vi "Check_with_Jump.vi"(0 "Current position":dbl[](array[numeric])=[0.0, 200.0, 40.0] format="%.2f", 1 "Traverse Name":string, 3 "Simulate/Run":T2=enum."Run VI", 5 "New Position":dbl[](array[numeric])=[0.0, 100.0, 40.0] format="%.2f", 7 "Probe Support":T1=[{"Max"=10.0, "Min"=-10.0}, {"Max"=10.0, "Min"=-10.0}, {"Max"=200.0, "Min"=0.0}] {"Min" format="%#.1f"; "Max" format="%#.1f"}, 9 "Entire Space":T1=[{"Max"=500.0, "Min"=-500.0}, {"Max"=1000.0, "Min"=-1000.0}, {"Max"=700.0, "Min"=0.0}] {"Min" format="%#.1f"; "Max" format="%#.1f"}, 11 "Probe Volume":T1=[{"Max"=10.0, "Min"=-10.0}, {"Max"=10.0, "Min"=-10.0}, {"Max"=200.0, "Min"=0.0}] {"Min" format="%#.1f"; "Max" format="%#.1f"}, 13 "Exclude Array":T3[](array[typedef])=[{"Sizes"=[{"Max"=1000.0, "Min"=-1000.0}, {"Max"=1000.0, "Min"=-1000.0}, {"Max"=20.0, "Min"=0.0}], "Name"="Roughness Elements", "Exclude Type"=enum."Allow only vertical moves"}, {"Sizes"=[{"Max"=50.0, "Min"=-50.0}, {"Max"=50.0, "Min"=-50.0}, {"Max"=220.0, "Min"=-0.0}], "Name"="B204", "Exclude Type"=enum."Exclude completely"}] {"Sizes"."Min" format="%#.1f"; "Sizes"."Max" format="%#.1f"}, 14 "Model       Roll      Pitch       Yaw (deg)":dbl[](array[numeric]) format="%#.2f") -> (4 "Error Comments":string, 10 "Steps":dbl[][](array[numeric])=[[0.0, 200.0, 40.0]] format="%.2f")   [LabVIEW 2013]
uses:
  Box_size.ctl
  Exclude_cluster.ctl
  Exclusion_type.ctl
  Controls/User_Specific_mode.ctl
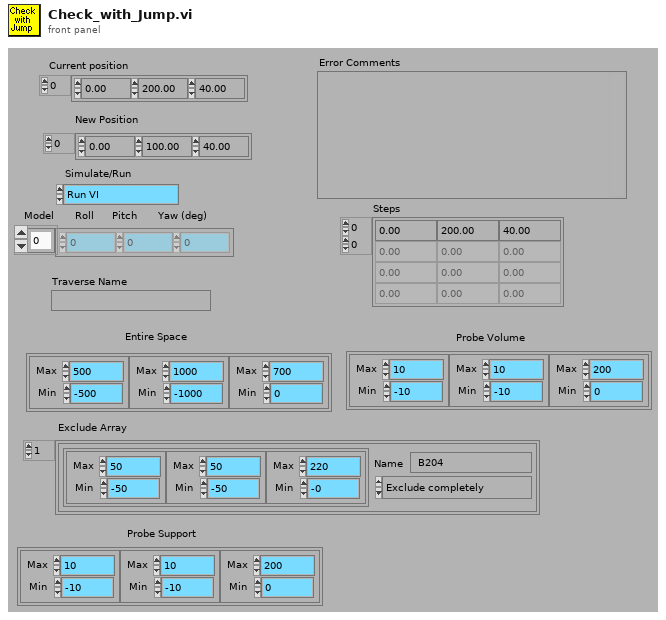
[diagram p1: front panel]
types:
  T1 = typedef "Box_size.ctl" = cluster{"Max":dbl, "Min":dbl}[]
  T2 = typedef "User_Specific_mode.ctl" = enum16{"Check VI only", "Run VI"}
  T3 = typedef "Exclude_cluster.ctl" = cluster{"Sizes":T1, "Name":string, "Exclude Type":T4}
  T4 = typedef "Exclusion_type.ctl" = enum16{"Exclude completely", "Allow only vertical moves"}
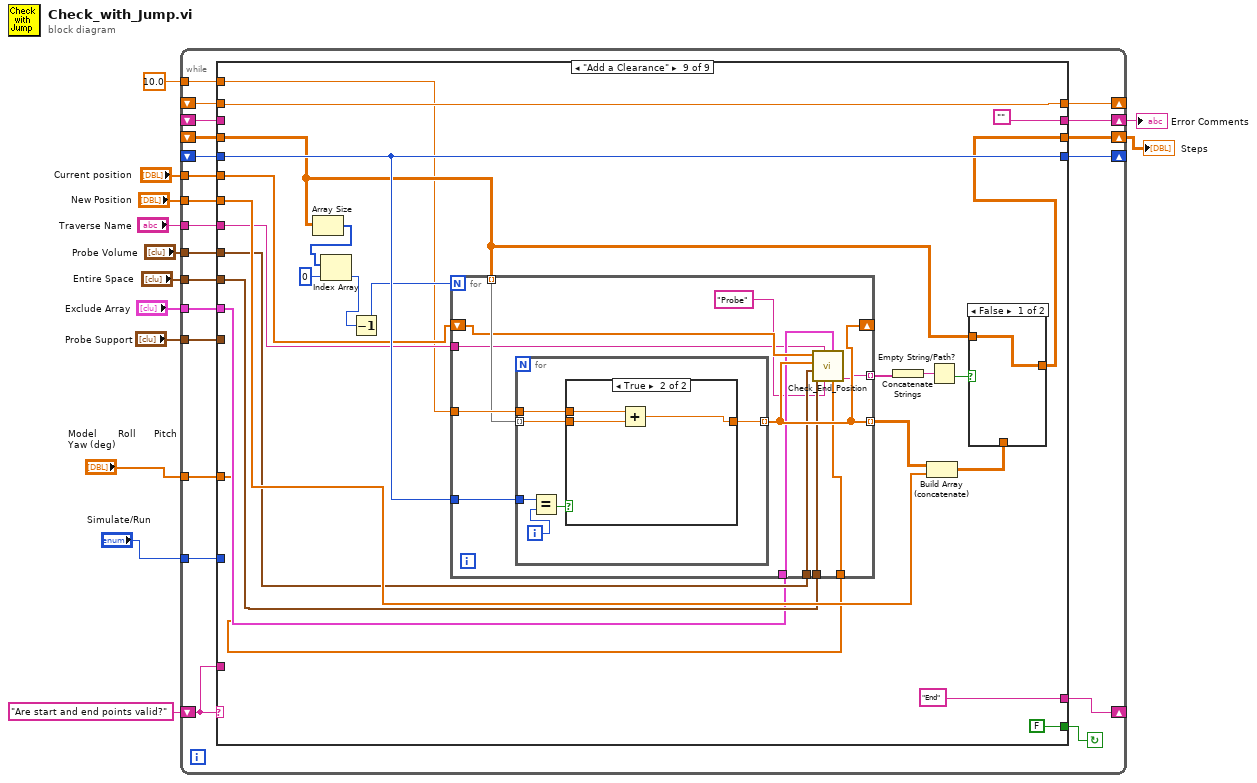
[diagram p0: block diagram]
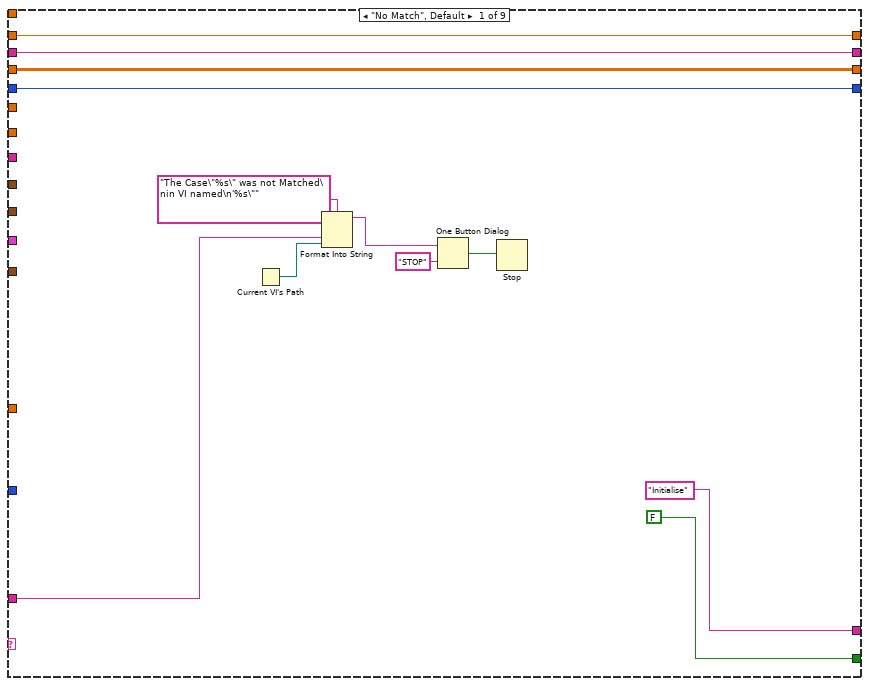
[diagram p2: hidden frame]
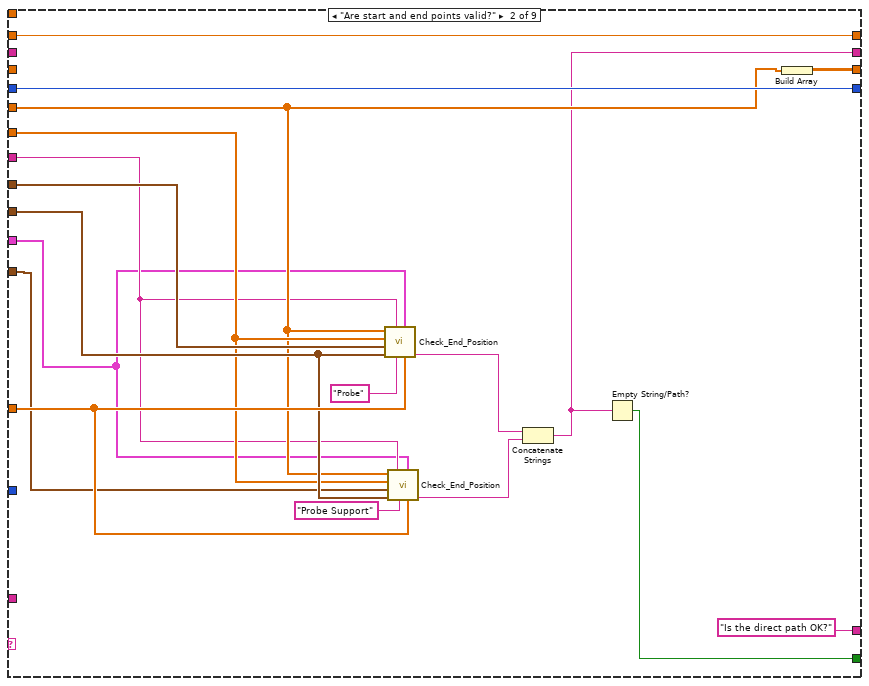
[diagram p3: hidden frame]
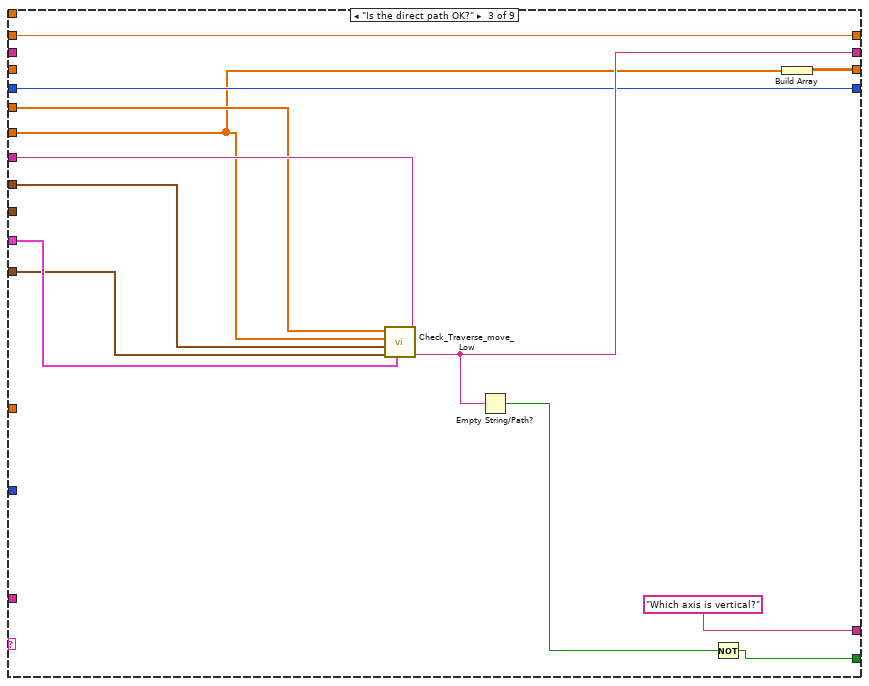
[diagram p4: hidden frame]
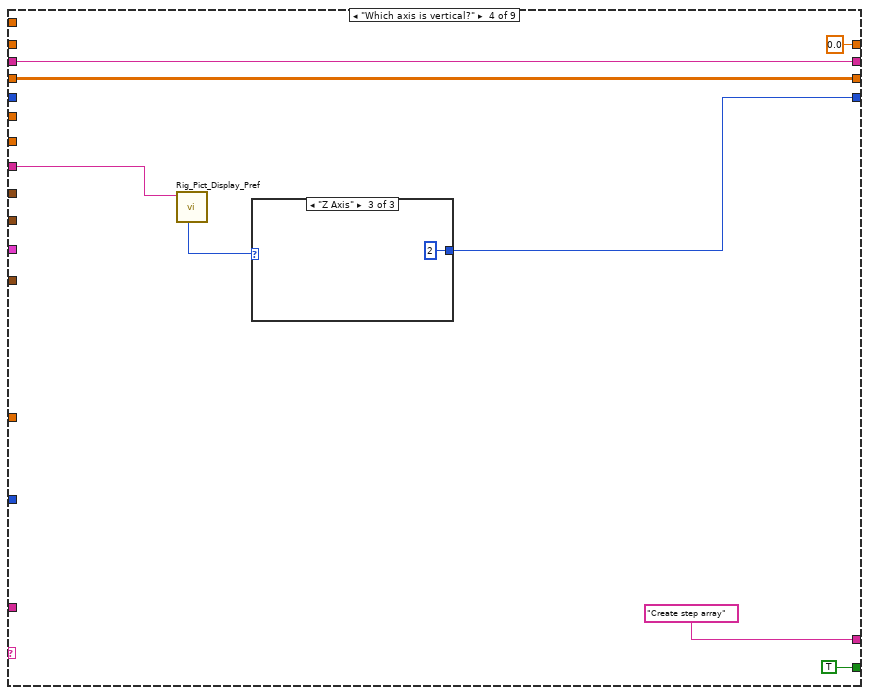
[diagram p5: hidden frame]
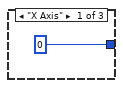
[diagram p6: hidden frame]
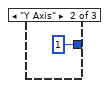
[diagram p7: hidden frame]
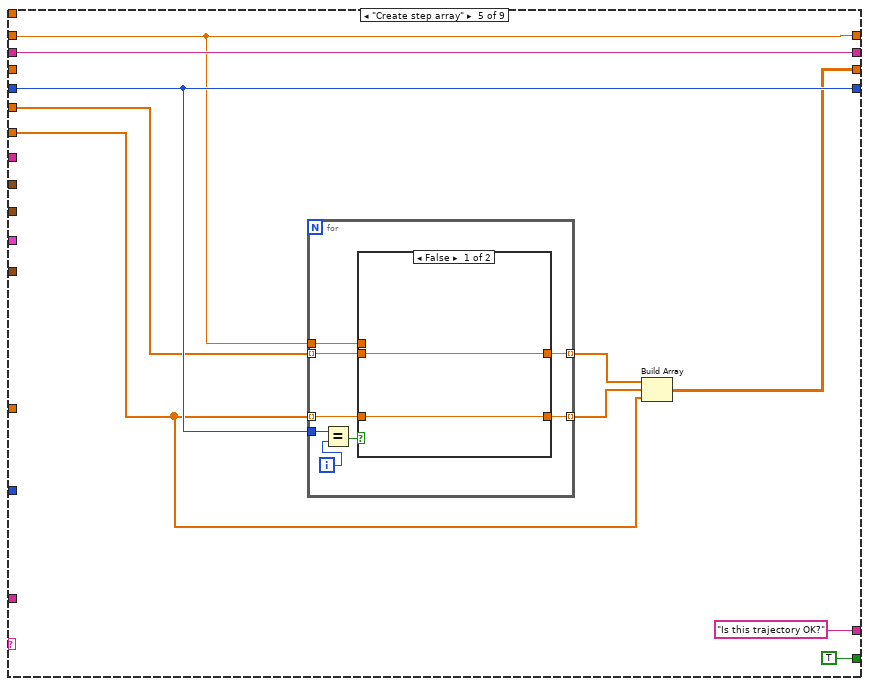
[diagram p8: hidden frame]
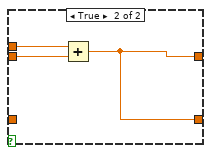
[diagram p9: hidden frame]
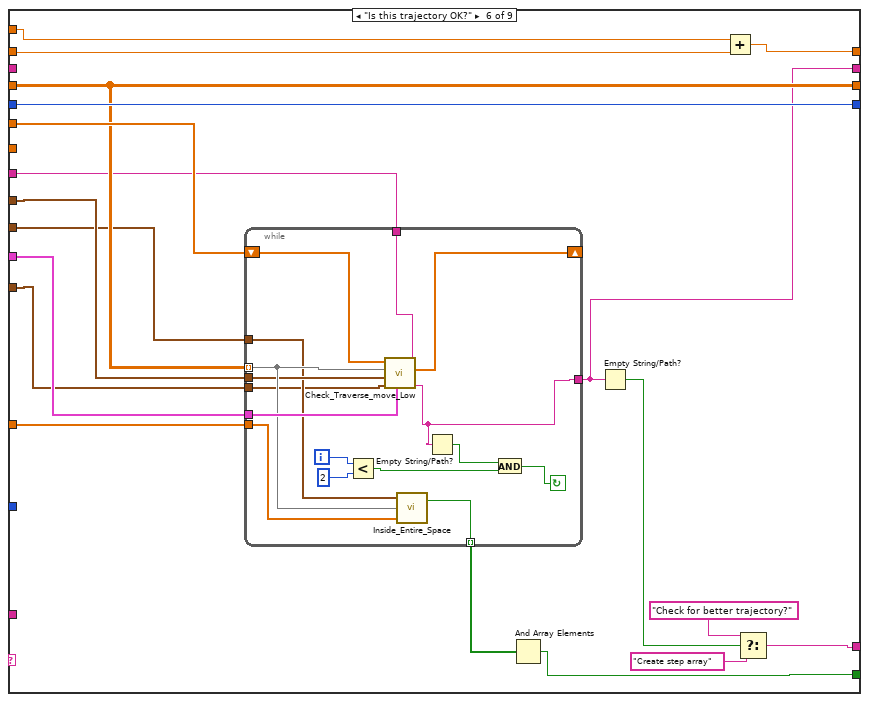
[diagram p10: hidden frame]
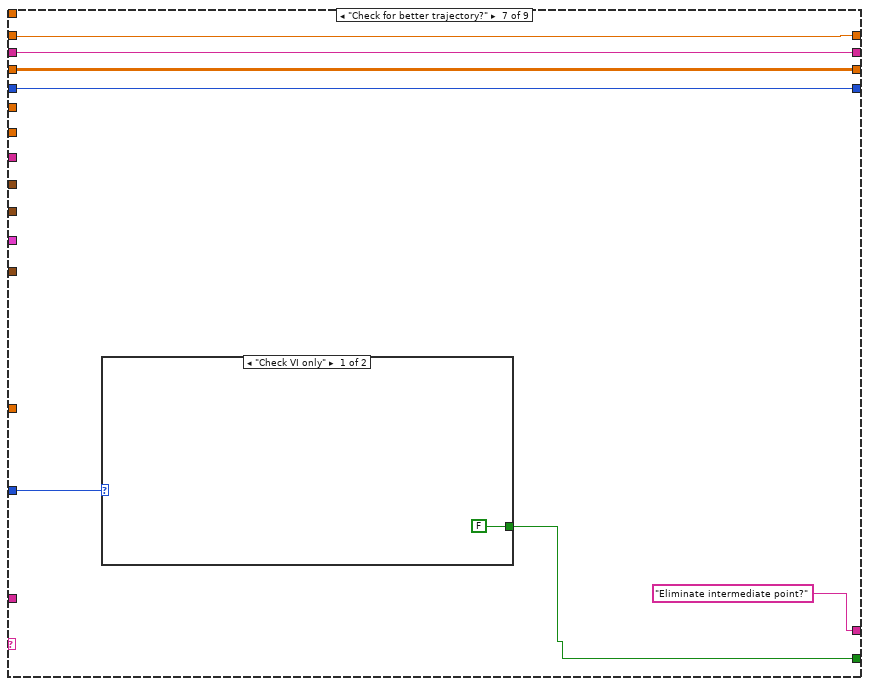
[diagram p11: hidden frame]
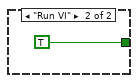
[diagram p12: hidden frame]
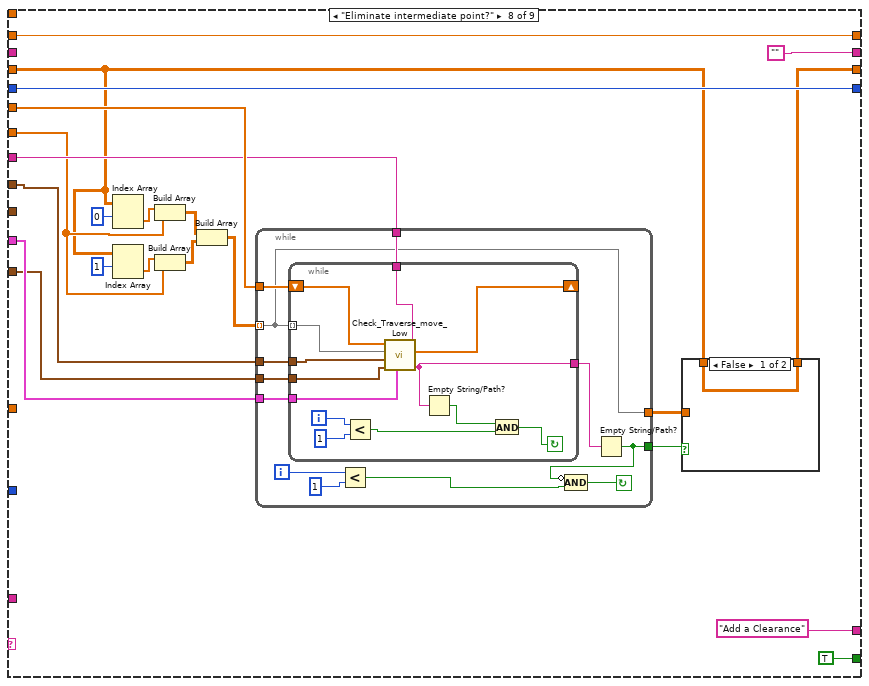
[diagram p13: hidden frame]
diagram:
  n1 = while {
    shift-left: "Are start and end points valid?" -> [w33]
    shift-right: [w34] -> _
    shift-right: [w30] -> w5
    shift-left: _ -> [w31]
    shift-right: [w29] -> w6
    shift-left: _ -> [w28]
    tunnel: "Current position" -> [w27]
    tunnel: "New Position" -> [w26]
    tunnel: "Probe Volume" -> [w25]
    tunnel: "Entire Space" -> [w24]
    tunnel: "Exclude Array" -> [w23]
    tunnel: "Traverse Name" -> [w22]
    shift-right: [w21] -> _
    shift-left: _ -> [w20]
    shift-right: [w19] -> _
    shift-left: _ -> [w18]
    tunnel: 10.0 -> [w17]
    tunnel: "Simulate/Run" -> [w16]
    tunnel: "Model       Roll      Pitch       Yaw (deg)" -> [w15]
    tunnel: "Probe Support" -> [w14]
    stop <- w32 continue-if-true
    n2 = case shown="\"Add a Clearance\"" w33 {
      tunnel: [FALSE w61 w69 TRUE TRUE w113 w147 TRUE FALSE] -> w32
      tunnel: ["Initialise" "Is the direct path OK?" "Which axis is vertical?" "Create step array" "Is this trajectory OK?" w123 "Eliminate intermediate point?" "Add a Clearance" "End"] -> w34
      tunnel: w33 -> [w41 _ _ _ _ _ _ _ _]
      tunnel: w31 -> [w38 _ _ w83 w97 _ w153 _ _]
      tunnel: [w38 w50 w73 w83 w97 w120 w153 "" ""] -> w30
      tunnel: [w37 w62 w71 w84 w90 w128 w150 w163 w213] -> w29
      tunnel: w28 -> [w37 _ _ w84 _ w128 w150 w161 w212]
      tunnel: w27 -> [_ w54 w72 _ w94 w129 _ w176 w218]
      tunnel: w26 -> [_ w55 w66 _ w91 _ _ w168 w219]
      tunnel: w25 -> [_ w63 w76 _ _ w127 _ w175 w211]
      tunnel: w24 -> [_ w57 _ _ _ w115 _ _ w210]
      tunnel: w23 -> [_ w47 w75 _ _ w126 _ w174 w209]
      tunnel: w22 -> [_ w53 w74 w82 _ w125 _ w173 w208]
      tunnel: [w36 w60 w68 w80 w95 w130 w152 w177 w226] -> w21
      tunnel: w20 -> [w36 w60 w68 _ w95 w130 w152 w177 w226]
      tunnel: [w35 w59 w67 0.0 w89 w117 w151 w160 w224] -> w19
      tunnel: w18 -> [w35 w59 w67 _ w89 w119 w151 w160 w224]
      tunnel: w17 -> [_ _ _ _ _ w118 _ _ w206]
      tunnel: w16 -> [_ _ _ _ _ _ w149 _ _]
      tunnel: w15 -> [_ w58 _ _ _ w116 _ _ w205]
      tunnel: w14 -> [_ w56 w65 _ _ w112 _ w156 _]
      frame "No Match", Default {
        n3 = Current VI's Path() -> (path=w40:path)
        n4 = Format Into String(format string="The Case\"%s\" was not Matched\nin VI named\n'%s\"" ("Format String"), w41, w40) -> (resulting string=w44:string)  [unwired: 2 in, 1 out]
        n5 = One Button Dialog(message=w44, button name ("OK")="STOP") -> (true=w42:bool)
        n6 = Stop(stop? (T)=w42) -> ()
      }
      frame "Are start and end points valid?" {
        n7 = call "Check_End_Position.vi"("Model       Roll      Pitch       Yaw (deg)"=w58, "Exclude Array"=w47, "Volume Name"="Probe", "Traverse Name"=w53, "Entire Space"=w57, "Probe Volume"=w63, "New Position"=w55, "Current position"=w54) -> ("Error Comments"=w49:string)  [unwired: 3 in]
        n8 = call "Check_End_Position.vi"("Model       Roll      Pitch       Yaw (deg)"=w58, "Exclude Array"=w47, "Volume Name"="Probe Support", "Traverse Name"=w53, "Entire Space"=w57, "Probe Volume"=w56, "New Position"=w55, "Current position"=w54) -> ("Error Comments"=w48:string)  [unwired: 3 in]
        n9 = Concatenate Strings(w49, w48) -> (w50:string)
        n10 = Empty String/Path?(string/path=w50) -> (empty?=w61:bool)
        n11 = Build Array(w54) -> (w62:dbl[][])
      }
      frame "Is the direct path OK?" {
        n12 = call "Check_Traverse_move_Low.vi"("Traverse Name"=w74, "Exclude Array"=w75, "Probe Support"=w65, "Probe Volume"=w76, "New Position"=w66, "Current position"=w72) -> ("Error Comments"=w73:string)  [unwired: 1 in, 2 out]
        n13 = Empty String/Path?(string/path=w73) -> (empty?=w70:bool)
        n14 = Not(x=w70) -> (.not. x?=w69:bool)
        n15 = Build Array(w66) -> (w71:dbl[][])
      }
      frame "Which axis is vertical?" {
        n16 = call "Rig_Pict_Display_Pref.vi"("Traverse Name"=w82) -> ("Which Axis is vertical?"=w81:enum16{"X Axis", "Y Axis", "Z Axis"})  [unwired: 7 out]
        n17 = case shown="\"Z Axis\"" w81 {
          tunnel: [0 1 2] -> w80
          frame "X Axis" {
          }
          frame "Y Axis" {
          }
          frame "Z Axis" {
          }
        }
      }
      frame "Create step array" {
        n18 = for {
          tunnel: w89 -> [w106]
          tunnel: w95 -> [w103]
          tunnel: w94 -> [w102] mode=indexing
          tunnel: [w101] -> w93 mode=indexing
          tunnel: w91 -> [w100] mode=indexing
          tunnel: [w99] -> w92 mode=indexing
          i -> [w105]
          n19 = Equal?(x=w103, y=w105) -> (x = y?=w104:bool)
          n20 = case shown="False" w104 {
            tunnel: w106 -> [_ w111]
            tunnel: w102 -> [w108 w110]
            tunnel: [w108 w109] -> w101
            tunnel: w100 -> [w107 _]
            tunnel: [w107 w109] -> w99
            frame False {
            }
            frame True {
              n21 = Add(x=w111, y=w110) -> (x+y=w109:dbl)
            }
          }
        }
        n22 = Build Array(w93, w92, w91) -> (w90:dbl[][])
      }
      frame "Is this trajectory OK?" {
        n23 = while {
          shift-right: [w140] -> _
          shift-left: w129 -> [w141]
          tunnel: w128 -> [w136] mode=indexing
          tunnel: w127 -> [w135]
          tunnel: w126 -> [w138]
          tunnel: w125 -> [w139]
          tunnel: [w137] -> w120
          tunnel: w116 -> [w134]
          tunnel: w115 -> [w132]
          tunnel: [w133] -> w114 mode=indexing
          tunnel: w112 -> [w131]
          i -> [w142]
          stop <- w143 continue-if-true
          n24 = Less?(x=w142, y=2 ("x")) -> (x < y?=w144:bool)
          n25 = call "Check_Traverse_move_Low.vi"("Traverse Name"=w139, "Exclude Array"=w138, "Probe Support"=w131, "Probe Volume"=w135, "New Position"=w136, "Current position"=w141) -> ("Error Comments"=w137:string, "Position At Crash"=w140:dbl[])  [unwired: 1 in, 1 out]
          n26 = call "Inside_Entire_Space.vi"("Model       Roll      Pitch       Yaw (deg)"=w134, "Current Position"=w136, "Envelope"=w132) -> ("Box Inside"=w133:bool)  [unwired: 1 out]
          n27 = Empty String/Path?(string/path=w137) -> (empty?=w145:bool)
          n28 = And(x=w145, y=w144) -> (x .and. y?=w143:bool)
        }
        n29 = And Array Elements(Boolean array=w114) -> (logical AND=w113:bool)
        n30 = Empty String/Path?(string/path=w120) -> (empty?=w124:bool)
        n31 = Add(x=w118, y=w119) -> (x+y=w117:dbl)
        n32 = Select(t="Check for better trajectory?", s=w124, f="Create step array") -> (s? t:f=w123:string)
      }
      frame "Check for better trajectory?" {
        n33 = case shown="\"Check VI only\"" w149 {
          tunnel: [FALSE TRUE] -> w147
          frame "Check VI only" {
          }
          frame "Run VI" {
          }
        }
      }
      frame "Eliminate intermediate point?" {
        n34 = Index Array(array=w161, index (row)=0) -> (element=w170:dbl[])  [unwired: 1 in]
        n35 = Index Array(array=w161, index (row)=1) -> (element=w169:dbl[])  [unwired: 1 in]
        n36 = Build Array(w170, w168) -> (w167:dbl[][])
        n37 = Build Array(w169, w168) -> (w166:dbl[][])
        n38 = Build Array(w167, w166) -> (w165:dbl[][][])
        n39 = while {
          tunnel: w176 -> [w191]
          tunnel: w175 -> [w190]
          tunnel: w174 -> [w189]
          tunnel: w173 -> [w188]
          tunnel: w165 -> [w181] mode=indexing
          tunnel: [w182] -> w164
          tunnel: [w181] -> w162
          tunnel: w156 -> [w180]
          i -> [w185]
          stop <- w183 continue-if-true
          n40 = while {
            shift-right: [w200] -> _
            shift-left: w191 -> [w204]
            tunnel: w190 -> [w203]
            tunnel: w189 -> [w202]
            tunnel: w188 -> [w201]
            tunnel: [w194] -> w187
            tunnel: w181 -> [w193] mode=indexing
            tunnel: w180 -> [w192]
            i -> [w199]
            stop <- w195 continue-if-true
            n41 = Less?(x=w199, y=1 ("x")) -> (x < y?=w196:bool)
            n42 = call "Check_Traverse_move_Low.vi"("Traverse Name"=w201, "Exclude Array"=w202, "Probe Support"=w192, "Probe Volume"=w203, "New Position"=w193, "Current position"=w204) -> ("Error Comments"=w194:string, "Position At Crash"=w200:dbl[])  [unwired: 1 in, 1 out]
            n43 = Empty String/Path?(string/path=w194) -> (empty?=w197:bool)
            n44 = And(x=w197, y=w196) -> (x .and. y?=w195:bool)
          }
          n45 = Less?(x=w185, y=1 ("x")) -> (x < y?=w184:bool)
          n46 = Empty String/Path?(string/path=w187) -> (empty?=w182:bool)
          n47 = Compound Arithmetic op=AND(invert w182, w184) -> (w183:bool)
        }
        n48 = case shown="False" w164 {
          tunnel: [w178 w179] -> w163
          tunnel: w162 -> [_ w179]
          tunnel: w161 -> [w178 _]
          frame False {
          }
          frame True {
          }
        }
      }
      frame "Add a Clearance" {
        n49 = Array Size(array=w212) -> (size(s)=w223:i32[])
        n50 = Index Array(array=w223, index=0) -> (element=w221:i32)
        n51 = Decrement(x=w221) -> (x-1=w220:i32)
        n52 = for {
          N: w220 -> [_]
          tunnel: w226 -> [w242]
          tunnel: [w238] -> w225 mode=indexing
          tunnel: w206 -> [w241]
          tunnel: w212 -> [w240] mode=indexing
          shift-right: [w238] -> _
          shift-left: w218 -> [w239]
          tunnel: [w237] -> w217 mode=indexing
          tunnel: w211 -> [w236]
          tunnel: w210 -> [w235]
          tunnel: w209 -> [w234]
          tunnel: w208 -> [w233]
          tunnel: w205 -> [w232]
          n53 = for {
            tunnel: w241 -> [w248]
            tunnel: w242 -> [w245]
            tunnel: w240 -> [w244] mode=indexing
            tunnel: [w243] -> w238 mode=indexing
            i -> [w247]
            n54 = Equal?(x=w245, y=w247) -> (x = y?=w246:bool)
            n55 = case shown="True" w246 {
              tunnel: w248 -> [_ w252]
              tunnel: w244 -> [w249 w251]
              tunnel: [w249 w250] -> w243
              frame False {
              }
              frame True {
                n56 = Add(x=w252, y=w251) -> (x+y=w250:dbl)
              }
            }
          }
          n57 = call "Check_End_Position.vi"("Model       Roll      Pitch       Yaw (deg)"=w232, "Exclude Array"=w234, "Volume Name"="Probe", "Traverse Name"=w233, "Entire Space"=w235, "Probe Volume"=w236, "New Position"=w238, "Current position"=w239) -> ("Error Comments"=w237:string)  [unwired: 3 in]
        }
        n58 = Concatenate Strings(w217) -> (w216:string)
        n59 = Build Array (concatenate)(w225, w219) -> (w214:dbl[][])
        n60 = Empty String/Path?(string/path=w216) -> (empty?=w215:bool)
        n61 = case shown="False" w215 {
          tunnel: w214 -> [_ w230]
          tunnel: [w229 w230] -> w213
          tunnel: w212 -> [w229 _]
          frame False {
          }
          frame True {
          }
        }
      }
    }
  }
  "Error Comments" <- w5
  "Steps" <- w6
